vi "Test Initialize.vi"(0 "Test Template in":refnum<class "niDTS Calibration Cal IsNeeded RF Test.lvclass">, 11 "error in (no error)":errorcluster) -> (4 "Test Template out":refnum<class "niDTS Calibration Cal IsNeeded RF Test.lvclass">, 15 "error out":errorcluster)   [LabVIEW 2015, in "niDTS Utilities.lvlib" / "niDTS Calibration Cal IsNeeded RF Test.lvclass"]
uses:
  niDTS Calibration Cal IsNeeded RF Test.lvclass
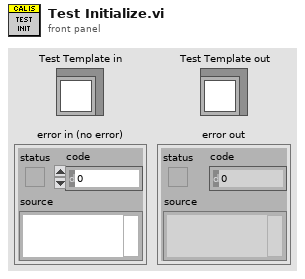
[diagram p1: front panel]
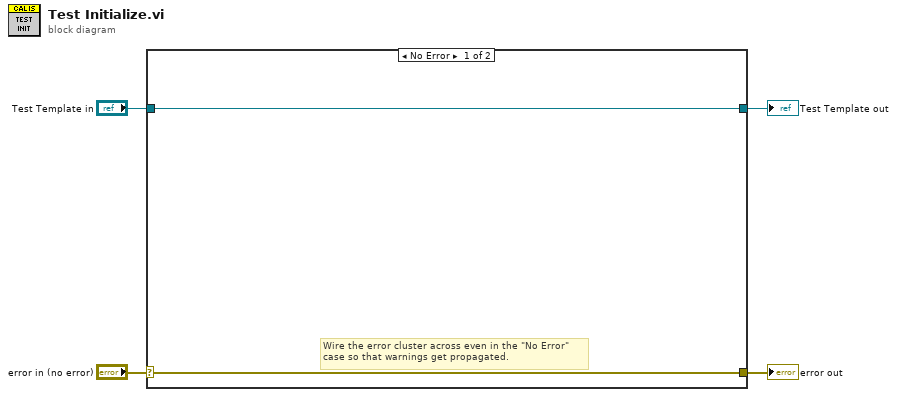
[diagram p0: block diagram]
diagram:
  n1 = case shown="No Error" "error in (no error)" {
    selector: "error in (no error)" -> [w5 w8]
    tunnel: [w5 w8] -> w3
    tunnel: [w6 w7] -> w1
    tunnel: "Test Template in" -> [w6 w7]
    frame No Error {
      # "Wire the error cluster across even in the \"No Error\"\ncase so that warnings get propagated."
    }
    frame Error {
    }
  }
  "error out" <- w3
  "Test Template out" <- w1
